vi "Read Model Number.vi"(7 "Unit ID (A)":string="A", 8 "error in":errorcluster, 11 "VISA Session In":refnum<visa-resource-name>="Alicat") -> (0 "error out":errorcluster, 2 "Model Number":string, 3 "VISA Session Out":refnum<visa-resource-name>)   [LabVIEW 2015]
doc: "Reads the model number of the device from the stored manufacturer's data query."
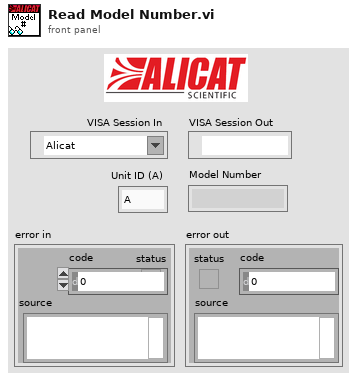
[diagram p1: front panel]
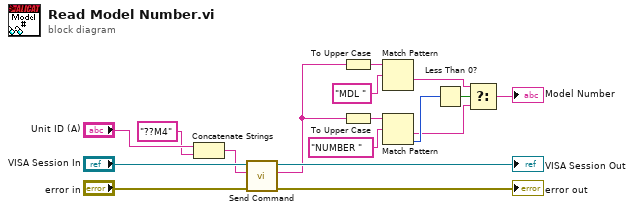
[diagram p0: block diagram]
diagram:
  n1 = Concatenate Strings("Unit ID (A)", "??M4") -> (w11:string)
  n2 = call "Send Command.vi"("error in"="error in", "Command"=w11, "VISA Session In"="VISA Session In") -> ("error out"=→"error out":errorcluster, "Response"=w6:string, "VISA Session Out"=→"VISA Session Out":refnum<visa-resource-name>)  [unwired: 6 in]
  n3 = To Upper Case(1:w6) -> (0:w8:string)
  n4 = To Upper Case(1:w6) -> (0:w15:string)
  n5 = Match Pattern(string=w8, regular expression="MDL ") -> (after substring=w3:string)  [unwired: 1 in, 3 out]
  n6 = Match Pattern(string=w15, regular expression="NUMBER ") -> (after substring=w2:string, offset past match=w5:i32)  [unwired: 1 in, 2 out]
  n7 = Less Than 0?(x=w5) -> (x < 0?=w4:bool)
  n8 = Select(t=w3, s=w4, f=w2) -> (s? t:f=→"Model Number":string)
